vi "Modulation-Create (contin).vi"(8 "error in (no error)":errorcluster, 9 "sampling info":T5={"Fs"=1000.0, "N"=1000} {"Fs" format="%.2p"}, 10 "Old":T1={"SAM"={"Active"=FALSE, "Frequency (Hz)"=0.0, "Depth"=0.0, "Init Phase (cycles)"=0.0, "phase (degrees)"=0.0, "Asynch"=FALSE}, "BAM"={"Frequency (Hz)"=0.0, "Duration (ms)"=0.0, "Ramp (ms)"=0.0}, "Mod Type"=enum."Sinusoidal"}, 11 "New":T1={"SAM"={"Active"=FALSE, "Frequency (Hz)"=0.0, "Depth"=0.0, "Init Phase (cycles)"=0.0, "phase (degrees)"=0.0, "Asynch"=FALSE}, "BAM"={"Frequency (Hz)"=0.0, "Duration (ms)"=0.0, "Ramp (ms)"=0.0}, "Mod Type"=enum."Sinusoidal"}) -> (0 "error out":errorcluster, 2 "Modulation":dbl[](array[numeric]), 3 "Modul Out":T1={"SAM"={"Active"=FALSE, "Frequency (Hz)"=0.0, "Depth"=0.0, "Init Phase (cycles)"=0.0, "phase (degrees)"=0.0, "Asynch"=FALSE}, "BAM"={"Frequency (Hz)"=0.0, "Duration (ms)"=0.0, "Ramp (ms)"=0.0}, "Mod Type"=enum."Sinusoidal"})   [LabVIEW 2015]
doc: "Takes a generic waveform description and returns a token of the specific waveform."
uses:
  Controls/Modulation XCtl/Modulation Data.ctl
  SAM VIs/SAM Params.ctl
  BAM VIs/BAM Params.ctl
  Controls/Modulation XCtl/Modulation Type.ctl
  Controls/Typedefs/Sampling Info.ctl
  <vilib>/Analysis/1siggen.llb/Ramp Pattern by Samples.vi
  <vilib>/Analysis/NI_AALBase.lvlib
  Controls/Modulation XCtl/Modulation.xctl
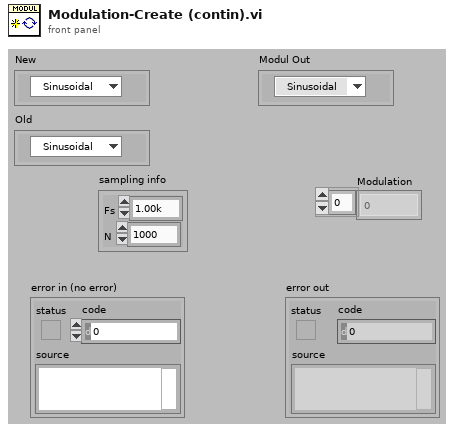
[diagram p1: front panel]
types:
  T1 = typedef "Modulation.xctl/Modulation Data.ctl" = cluster{"SAM":T2, "BAM":T3, "Mod Type":T4}
  T2 = typedef "SAM Params.ctl" = cluster{"Active":bool, "Frequency (Hz)":dbl, "Depth":dbl, "Init Phase (cycles)":dbl, "phase (degrees)":dbl, "Asynch":bool}
  T3 = typedef "BAM Params.ctl" = cluster{"Frequency (Hz)":dbl, "Duration (ms)":dbl, "Ramp (ms)":dbl}
  T4 = typedef "Modulation Type.ctl" = enum16{"OFF", "Sinusoidal", "Bursted"}
  T5 = typedef "Sampling Info.ctl" = cluster{"Fs":dbl, "N":i32}
  T6 = typedef "Tone Params.ctl" = cluster{"Frequency (kHz)":dbl, "Last Freq":dbl, "Last Phase":dbl}
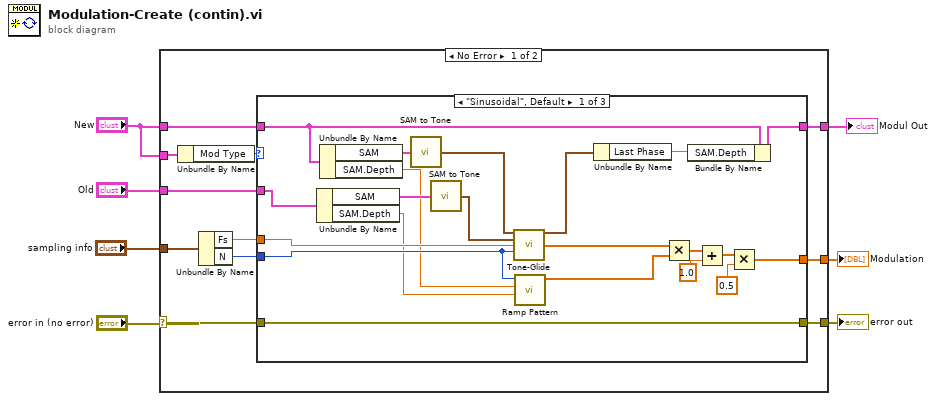
[diagram p0: block diagram]
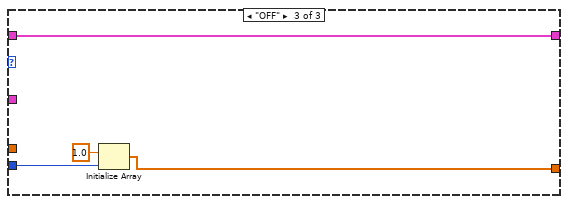
[diagram p3: hidden frame]
diagram:
  n1 = case shown="No Error" "error in (no error)" {
    selector: "error in (no error)" -> [w16 w47]
    tunnel: [w14 w47] -> w6
    tunnel: "New" -> [w18 _]
    tunnel: "New" -> [w15 w46]
    tunnel: [w13 _] -> w4
    tunnel: [w12 w46] -> w1
    tunnel: "sampling info" -> [w10 _]
    tunnel: "Old" -> [w8 _]
    frame No Error {
      n2 = Unbundle By Name(w18) -> ("Mod Type"=w17:T4)
      n3 = Unbundle By Name(w10) -> ("Fs"=w11:dbl, "N"=w9:i32)
      n4 = case shown="\"Sinusoidal\", Default" w17 {
        tunnel: w16 -> [w38 w40 _]
        tunnel: w11 -> [w37 _ _]
        tunnel: w9 -> [w23 _ w44]
        tunnel: w15 -> [w32 w41 w45]
        tunnel: [w38 w40 _] -> w14
        tunnel: [w24 _ w43] -> w13
        tunnel: [w39 w41 w45] -> w12
        tunnel: w8 -> [w36 _ _]
        frame "Sinusoidal", Default {
          n5 = Unbundle By Name(w36) -> ("SAM"=w33:T2, "SAM.Depth"=w21:dbl)
          n6 = Unbundle By Name(w32) -> ("SAM"=w31:T2, "SAM.Depth"=w22:dbl)
          n7 = call "SAM to Tone.vi"("SAM"=w31) -> ("Tone"=w30:T6)
          n8 = call "SAM to Tone.vi"("SAM"=w33) -> ("Tone"=w35:T6)
          n9 = call "Tone-Glide.vi"("New"=w30, "Old"=w35, "Fs (Hz)"=w37, "Npts"=w23) -> ("Params out"=w34:T6, "Y"=w25:dbl[])  [unwired: 10 in]
          n10 = call-poly <vilib>:"Ramp Pattern.vi"("start"=w21, "end"=w22, "samples"=w23) -> ("Ramp Pattern"=w20:dbl[])  [unwired: 7 in, 1 out]
          n11 = Unbundle By Name(w34) -> ("Last Phase"=w19:dbl)
          n12 = Multiply(x=w25, y=w20) -> (x*y=w29:dbl[])
          n13 = Bundle By Name(cluster=w32, "SAM.Depth"=w19) -> (w39:T1)
          n14 = Add(x=w29, y=1.0) -> (x+y=w27:dbl[])
          n15 = Multiply(x=w27, y=0.5) -> (x*y=w24:dbl[])
        }
        frame "Bursted" {
        }
        frame "OFF" {
          n16 = Initialize Array(1.0 ("element"), w44) -> (w43:dbl[])
        }
      }
    }
    frame Error {
    }
  }
  "error out" <- w6
  "Modulation" <- w4
  "Modul Out" <- w1
